vi "OA Write To File.vi"(10 "uiFileNameLen":u32, 11 "pcFileName":string) -> (3 "function return":u32)   [LabVIEW 2018, in "AndorSDK.lvlib"]
doc: "EXPNETTYPE unsigned int WINAPI OA_WriteToFile(const char * const pcFileName, unsigned int uiFileNameLen);"
uses:
  AndorSDK.lvlib
  ATMCD32D.dll
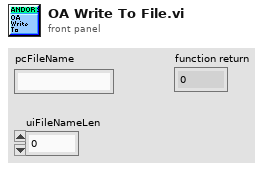
[diagram p1: front panel]
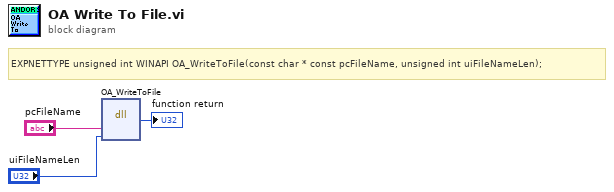
[diagram p0: block diagram]
diagram:
  # "EXPNETTYPE unsigned int WINAPI OA_WriteToFile(const char * const pcFileName, unsigned int uiFileNameLen);"
  n1 = dll-call lib="PTH2babs E\nPersönliches02 - Arbeit03-HiwijobsLabviewCodelibANDOR\tAndor SDK\nATMCD32D.*" fn="OA_WriteToFile"("pcFileName"="pcFileName", "uiFileNameLen"="uiFileNameLen") -> (→"function return":u32)  [unwired: 5 in, 2 out]
